vi "Get Biometry PD Parameter.vi"(8 "error in (no error)":errorcluster caption="错误输入（无错误）", 10 "condition":string, 11 "connection reference":T1) -> (0 "error out":errorcluster caption="错误输出", 2 "Data Output":string[][](array[string]), 3 "Measure_ID":i64[](array[numeric]))   [LabVIEW 2015, in "Utility VIs.lvlib"]
doc: "该模板用于创建子VI。"
uses:
  Utility VIs.lvlib
  <vilib>/addons/database/Connection.llb/Conn ObjectReference.ctl
  Database Processing/Database Processing.lvlib
  <vilib>/addons/database/NI_Database_API.lvlib
panel:
  # "Busy"
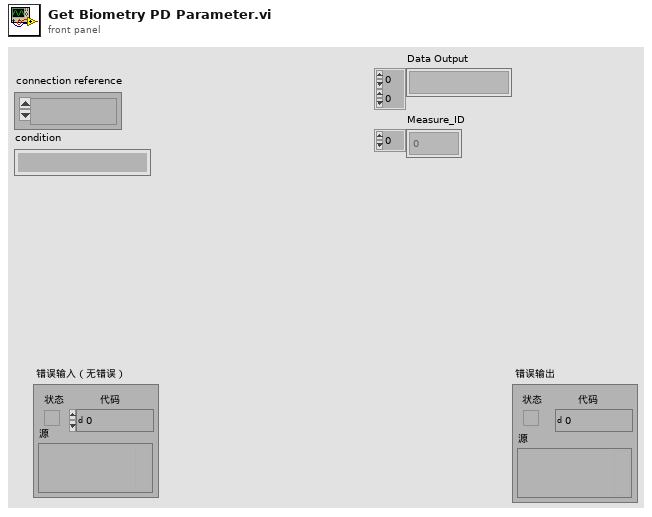
[diagram p1: front panel]
types:
  T1 = typedef "NI_Database_API.lvlib/Conn ObjectReference.ctl" = refnum<k1>
  T2 = typedef "Database Processing.lvlib/Biometry Attribute.ctl" = cluster{"Measure_ID":i64, "Measure_No":i64, "Ordinal":i64, "L_Or_R":string}
  T3 = typedef "Database Processing.lvlib/Biometry Parameter.ctl" = cluster{"Measure_ID":i64, "Central_Corneal_Thickness":sgl, "Anterior_Chamber_Depth":sgl, "Len_Thickness":sgl, "Retinal_Thickness":sgl, "Axis_Length":sgl, "Pupil_Diameter":sgl, "PCX":sgl, "PCY":sgl, "White_To_White":sgl, "ICX":sgl, "ICY":sgl, "Keratometric_flat":sgl, "Keratometric_steep":sgl, "Keratometric_Axis(flat)":sgl, "Keratometric_Axis(steep)":sgl, "Keratometric_AST":sgl}
  T4 = typedef "Database Processing.lvlib/Biometry State.ctl" = cluster{"Measure_ID":i64, "Central_Corneal_Thickness_State":string, "Anterior_Chamber_Depth_State":string, "Len_Thickness_State":string, "Retinal_Thickness_State":string, "Axis_Length_State":string, "Pupil_Diameter_State":string, "White_To_White_State":string, "Keratometric_flat_State":string, "Keratometric_steep_State":string}
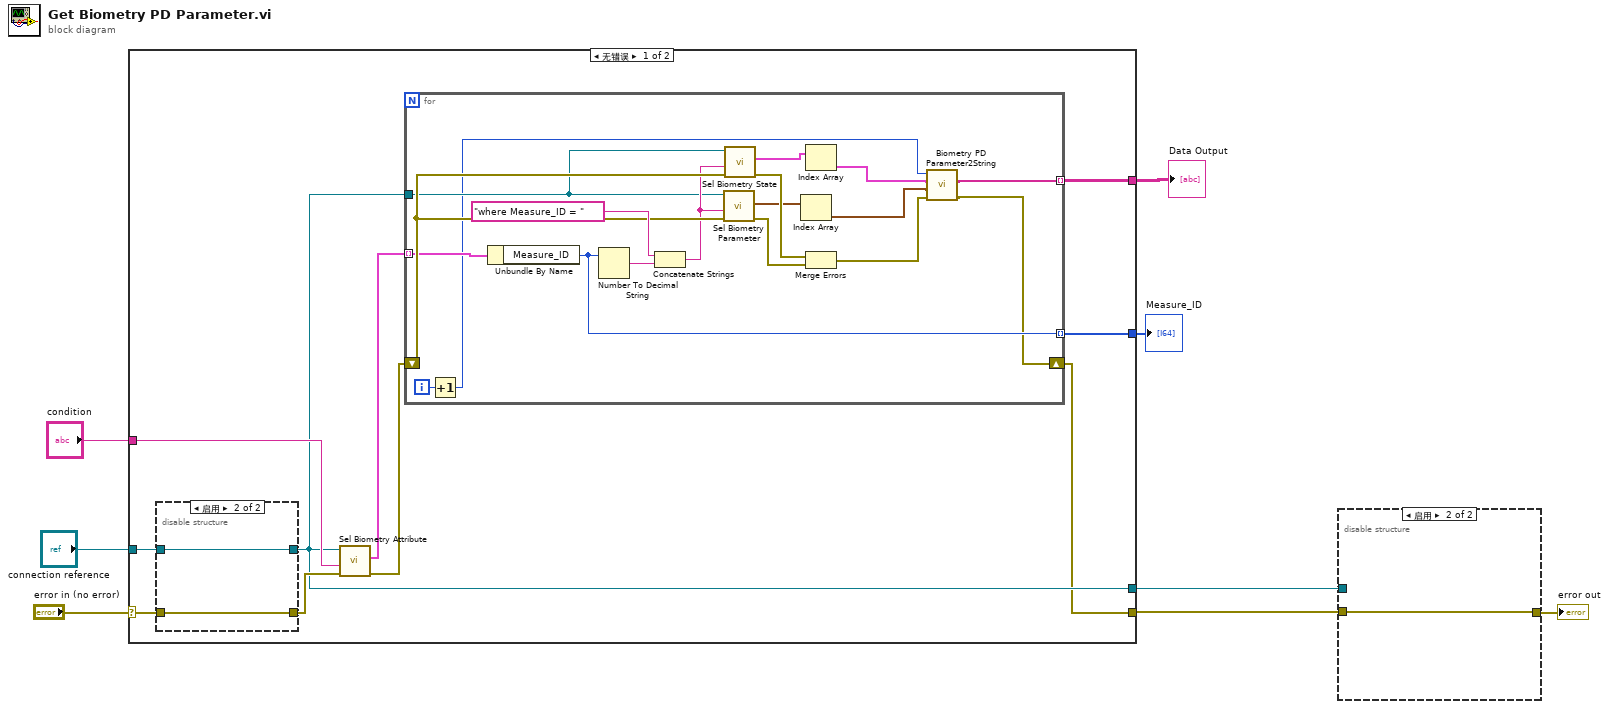
[diagram p0: block diagram]
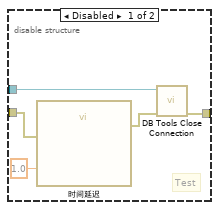
[diagram p2: hidden frame]
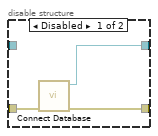
[diagram p3: hidden frame]
diagram:
  n1 = case shown="无错误" "error in (no error)" {
    selector: "error in (no error)" -> [w18 w43]
    tunnel: [w12 w43] -> w5
    tunnel: "connection reference" -> [w17 w42]
    tunnel: "condition" -> [w15 _]
    tunnel: [w13 w42] -> w3
    tunnel: [w10 _] -> w2
    tunnel: [w9 _] -> w1
    frame No Error {
      n2 = disable-structure shown="启用" {
        disable-tunnel: w18 -> [w39 w40]
        disable-tunnel: w17 -> [_ w41]
        disable-tunnel: [w38 w41] -> w13
        disable-tunnel: [w37 w40] -> w16
        frame Disabled {
          n3 = call "Connect Database.vi"("error in (no error)"=w39) -> ("error out"=w37:errorcluster, "connection reference"=w38:T1)  [unwired: 9 in]
        }
        frame Enabled {
        }
      }
      n4 = call "Sel Biometry Attribute.vi"("error in (no error)"=w16, "condition"=w15, "connection reference"=w13) -> ("error out"=w14:errorcluster, "Biometry Attribute"=w11:T2[])  [unwired: 7 in]
      n5 = for {
        tunnel: w13 -> [w32]
        shift-right: [w24] -> w12
        shift-left: w14 -> [w34]
        tunnel: w11 -> [w29] mode=indexing
        tunnel: [w19] -> w10 mode=indexing
        tunnel: [w26] -> w9 mode=indexing
        i -> [w25]
        n6 = Increment(x=w25) -> (x+1=w20:i32)
        n7 = Unbundle By Name(w29) -> ("Measure_ID"=w26:i64)
        n8 = Number To Decimal String(number=w26) -> (decimal integer string=w36:string)  [unwired: 1 in]
        n9 = Concatenate Strings("where Measure_ID = " ("字符串"), w36) -> (w33:string)
        n10 = call "Sel Biometry Parameter.vi"("error in (no error)"=w34, "condition"=w33, "connection reference"=w32) -> ("error out"=w30:errorcluster, "Biometry Parameter"=w27:T3[])  [unwired: 7 in]
        n11 = call "Sel Biometry State.vi"("error in (no error)"=w34, "condition"=w33, "connection reference"=w32) -> ("error out"=w31:errorcluster, "Biometry State"=w28:T4[])  [unwired: 7 in]
        n12 = Index Array(array=w27) -> (element=w22:T3)  [unwired: 1 in]
        n13 = Index Array(array=w28) -> (element=w21:T4)  [unwired: 1 in]
        n14 = Merge Errors(w31, w30) -> (w23:errorcluster)
        n15 = call "Biometry PD Parameter2String.vi"("error in (no error)"=w23, "Biometry Parameter"=w22, "Biometry State"=w21, "No"=w20) -> ("error out"=w24:errorcluster, "Data Output"=w19:string[])  [unwired: 6 in]
      }
    }
    frame Error {
    }
  }
  "Data Output" <- w2
  "Measure_ID" <- w1
  n16 = disable-structure shown="启用" {
    disable-tunnel: w5 -> [w46 w49]
    disable-tunnel: [w48 w49] -> w4
    disable-tunnel: w3 -> [w47 _]
    frame Disabled {
      # "Test"
      n17 = call "时间延迟"("error in (no error)"=w46, "Delay Time (s)"=1.0) -> ("error out"=w45:errorcluster)  [unwired: 9 in]
      n18 = call <vilib>:"DB Tools Close Connection.vi"("error in (no error)"=w45, "connection reference"=w47) -> ("error out"=w48:errorcluster)  [unwired: 5 in]
    }
    frame Enabled {
    }
  }
  "error out" <- w4
